vi "IOcard_singleAIConfig_Meilhaus.vi"(0 "Range":i32, 1 "Trigger Edge":T1(ring)=enum."Any", 2 "Trigger Type":T3(ring), 4 "Subdevice":i32, 5 "AI Reference":enum16{"Ground", "Differential"}(ring), 6 "Error input":errorcluster, 7 "Device":i32, 8 "Number of Channels":i32, 9 "Time Out":i32) -> (3 "Array":T2(array[cluster]))   [LabVIEW 2009]
uses:
  <userlib>/ME-iDS/ctls/meEnumTriggerChannel.ctl
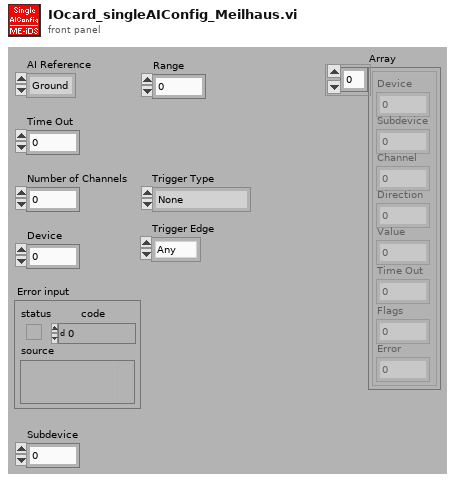
[diagram p1: front panel]
types:
  T1 = enum16{"None", "Above", "Below", "Entry", "Exit", "Rising", "Falling", "Any"}
  T2 = cluster{"Device":i32, "Subdevice":i32, "Channel":i32, "Direction":i32, "Value":i32, "Time Out":i32, "Flags":i32, "Error":i32}[]
  T3 = enum16{"None", "Software", "Threshold", "Window", "Edge", "Slope", "External Digital", "External Analog", "Pattern", "Timer", "Count", "Follow"}
  T4 = typedef "meEnumTriggerChannel.ctl" = enum16{"None", "Default", "Synchronous"}
  T5 = cluster{"Device":i32, "Subdevice":i32, "Channel":i32, "Direction":i32, "Value":i32, "Time Out":i32, "Flags":i32, "Error":i32}
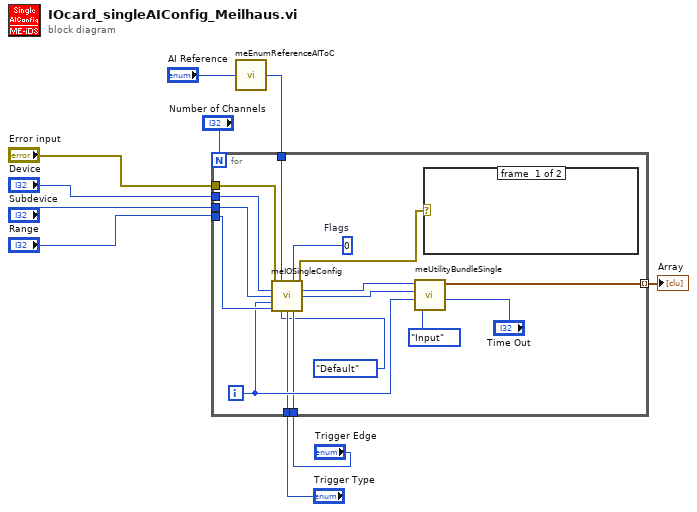
[diagram p0: block diagram]
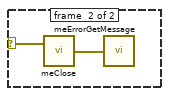
[diagram p2: hidden frame]
diagram:
  n1 = call <userlib>:"meEnumReferenceAIToC.vi"("AI Reference"="AI Reference") -> ("AI Reference Define Value"=w2:i32)
  n2 = for {
    N: "Number of Channels" -> [_]
    tunnel: "Error input" -> [w26]
    tunnel: "Device" -> [w25]
    tunnel: "Subdevice" -> [w24]
    tunnel: "Range" -> [w23]
    tunnel: w2 -> [w19]
    tunnel: "Trigger Type" -> [w18]
    tunnel: "Trigger Edge" -> [w17]
    tunnel: [w13] -> w4 mode=indexing
    i -> [w21]
    w22 = 0  # Flags
    n3 = call <userlib>:"meIOSingleConfig.vi"("error in (no error)"=w26, "Reference"=w19, "Flags"=w22, "Device"=w25, "Subdevice"=w24, "Channel"=w21, "Single Configuration"=w23, "Trigger Channel"=meEnumTriggerChannel."Default", "Trigger Type"=w18, "Trigger Edge"=w17) -> ("error out"=w20:errorcluster, "Device"=w16:i32, "Subdevice"=w15:i32)  [unwired: 3 in]
    n4 = call <userlib>:"meUtilityBundleSingle.vi"("Time Out"="Time Out", "Direction"=enum16{"Input", "Output"}."Input", "Channel"=w21, "Subdevice"=w15, "Device"=w16) -> ("Single Instruction"=w13:T5)  [unwired: 2 in]
    n5 = case shown="Fehler" w20 {
      selector: w20 -> [_ w28]
      frame #0 {
      }
      frame #1 {
        n6 = call <userlib>:"meClose.vi"("error in (no error)"=w28) -> ("error out"=w27:errorcluster)  [unwired: 1 in]
        n7 = call <userlib>:"meErrorGetMessage.vi"("error in (no error)"=w27) -> ()
      }
    }
  }
  "Array" <- w4
